vi "Calstruct_Write.vi"(8 "error in":errorcluster) -> (0 "error out":errorcluster, 3 "Return Code":i32)   [LabVIEW 2015]
doc: "This function will write the current local calibration structure back to the DSP storage (which is actually in the Cypress now)."
uses:
  ScannerDiagDLL.dll
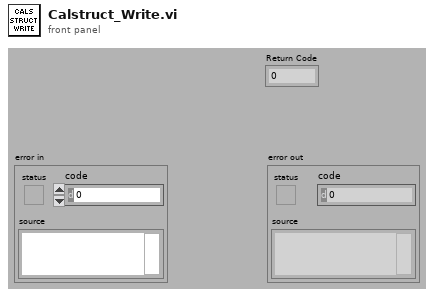
[diagram p1: front panel]
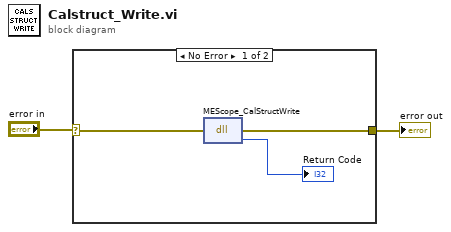
[diagram p0: block diagram]
diagram:
  n1 = case shown="No Error" "error in" {
    selector: "error in" -> [w5 w6]
    tunnel: [w4 w6] -> w1
    frame No Error {
      n2 = dll-call lib="C:/SNAPON/ModisEdge/TabletScope/Test Sequence/Code Modules/DLL/ScannerDiagDLL.dll" fn="MEScope_CalStructWrite"(error in=w5) -> (error out=w4:errorcluster, "return type"=→"Return Code":i32)  [unwired: 2 in, 1 out]
    }
    frame Error {
    }
  }
  "error out" <- w1
